vi "MultiplePatternMatch (SubVI).vi"(5 "Overlay Group":string, 6 "Label Colors":u32[](array[colorbox]), 7 "Learned Labels":string[](array[string]), 8 "error in (no error)":errorcluster, 9 "Match Labels":string[](array[string]), 10 "Match Results":T1(array[cluster]), 11 "Refnum in":T2) -> (0 "error out":errorcluster, 2 "Number of Matches":i32[](array[numeric]), 3 "Refnum out":T2)   [LabVIEW 2011]
uses:
  <vilib>/vision/Image Controls.llb/IMAQ Image.ctl
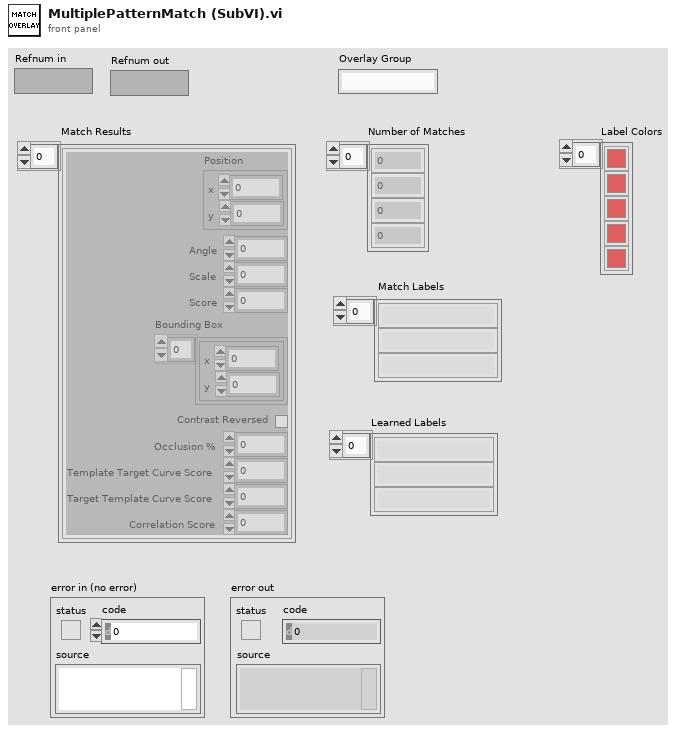
[diagram p1: front panel]
types:
  T1 = cluster{"Position":cluster{"x":sgl, "y":sgl}, "Angle":sgl, "Scale":sgl, "Score":sgl, "Bounding Box":cluster{"x":sgl, "y":sgl}[], "Contrast Reversed":bool, "Occlusion %":sgl, "Template Target Curve Score":sgl, "Target Template Curve Score":sgl, "Correlation Score":sgl}[]
  T2 = typedef "IMAQ Image.ctl" = refnum<image>
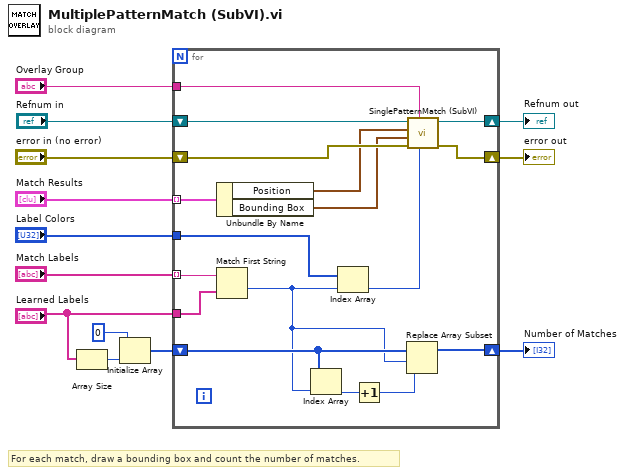
[diagram p0: block diagram]
diagram:
  # "For each match, draw a bounding box and count the number of matches."
  n1 = Array Size(array="Learned Labels") -> (size(s)=w4:i32)
  n2 = Initialize Array(0 ("x+1"), w4) -> (w6:i32[])
  n3 = for {
    shift-right: [w18] -> w1
    shift-left: "Refnum in" -> [w16]
    tunnel: "Match Results" -> [w30] mode=indexing
    tunnel: "Match Labels" -> [w29] mode=indexing
    shift-right: [w27] -> w2
    shift-left: w6 -> [w28]
    tunnel: "Learned Labels" -> [w24]
    shift-right: [w19] -> w11
    shift-left: "error in (no error)" -> [w20]
    tunnel: "Label Colors" -> [w22]
    tunnel: "Overlay Group" -> [w17]
    n4 = Unbundle By Name(w30) -> ("Position"=w15:cluster{"x":sgl, "y":sgl}, "Bounding Box"=w14:cluster{"x":sgl, "y":sgl}[])
    n5 = Match First String(2:w24, 3:w29) -> (0:w23:i32)  [unwired: 1 out]
    n6 = Index Array(array=w28, index=w23) -> (element=w26:i32)
    n7 = Index Array(array=w22, index=w23) -> (element=w21:u32)
    n8 = Increment(x=w26) -> (x+1=w25:i32)
    n9 = Replace Array Subset(array=w28, new element=w25, index=w23) -> (w27:i32[])
    n10 = call "SinglePatternMatch (SubVI).vi"("Color"=w21, "Group"=w17, "error in (no error)"=w20, "Bounding Box"=w14, "Position"=w15, "Refnum in"=w16) -> ("error out"=w19:errorcluster, "Refnum out"=w18:T2)  [unwired: 4 in]
  }
  "Refnum out" <- w1
  "Number of Matches" <- w2
  "error out" <- w11
